vi "실습 8-1.vi"() -> ()   [LabVIEW 2014]
uses:
  System.Windows.Forms
  System.Drawing
panel:
  out "Color":u32(colorbox) caption="색"
  out "Style":i32(ring) items=["Regular"=0, "Bold"=1, "Italic"=2, "Underline"=4, "Strikeout"=8]
  out "Size":sgl
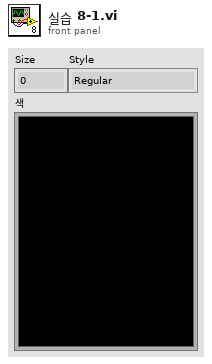
[diagram p1: front panel]
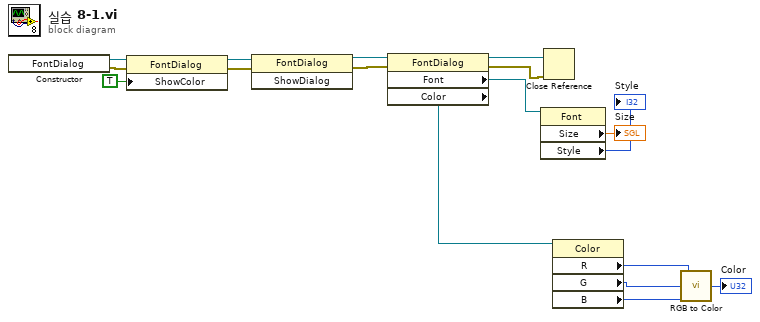
[diagram p0: block diagram]
diagram:
  n1 = constructor class="FontDialog"() -> (reference out=w5:refnum<k24>, error out=w3:errorcluster)  [unwired: 3 in, 1 out]
  n2 = property class="FontDialog"(reference=w5, error in=w3, "ShowColor"=TRUE) -> (reference out=w4:refnum<k24>, error out=w2:errorcluster)
  n3 = invoke class="FontDialog" method="ShowDialog"(reference=w4, error in=w2) -> (reference out=w17:refnum<k24>, error out=w16:errorcluster)  [unwired: 1 in, 1 out]
  n4 = property class="FontDialog"(reference=w17, error in=w16) -> (reference out=w15:refnum<k24>, error out=w14:errorcluster, "Font"=w13:refnum<k24>, "Color"=w10:refnum<k24>)
  n5 = property class="Font"(reference=w13) -> ("Size"=→"Size":sgl, "Style"=→"Style":i32)  [unwired: 1 in, 2 out]
  n6 = Close Reference(reference=w15, error in (no error)=w14) -> ()  [unwired: 1 out]
  n7 = property class="Color"(reference=w10) -> ("R"=w9:u8, "G"=w8:u8, "B"=w7:u8)  [unwired: 1 in, 2 out]
  n8 = call <vilib>:"RGB to Color.vi"("B"=w7, "G"=w8, "R"=w9) -> ("Color"=→"Color":u32)
